vi "MoveLineNumbers.vi"(10 "rows":refnum<vi>, 11 "code":refnum<vi>) -> (3 "rows":string)   [LabVIEW 2016, in "Code.xctl"]
uses:
  Code.xctl
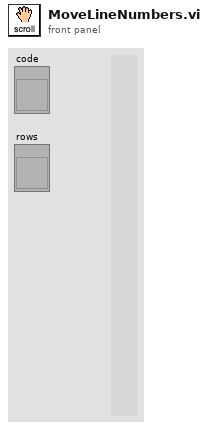
[diagram p1: front panel]
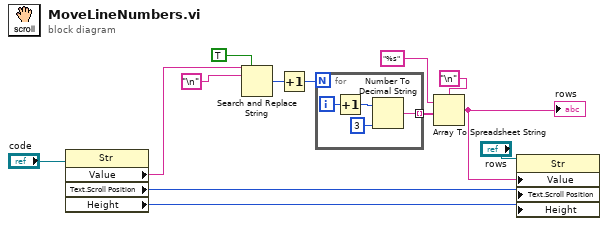
[diagram p0: block diagram]
diagram:
  n1 = property on="Property Node" class="Str"(reference="code") -> ("Value"=w3:string, "Text.Scroll Position"=w4:u32, "Height"=w8:u32)  [unwired: 1 in, 2 out]
  n2 = Search and Replace String(replace all?=TRUE ("replace all? (F)"), input string=w3, search string="\n") -> (number of replacements=w5:i32)  [unwired: 5 in, 3 out]
  n3 = Increment(x=w5) -> (x+1=w7:i32)
  n4 = for {
    N: w7 -> [_]
    tunnel: [w17] -> w6 mode=indexing
    i -> [w14]
    n5 = Increment(x=w14) -> (x+1=w16:i32)
    n6 = Number To Decimal String(number=w16, width (-)=i16 3) -> (decimal integer string=w17:string)
  }
  n7 = Array To Spreadsheet String(delimiter (Tab)="\n", array=w6, 3:"%s" ("format string")) -> (spreadsheet string=w1:string)
  "rows" <- w1
  n8 = property on="Property Node" class="Str"(reference="rows", "Value"=w1, "Text.Scroll Position"=w4, "Height"=w8) -> ()  [unwired: 1 in, 2 out]
